vi "FreqStep-Init.vi"(0 "Fs (Hz)":dbl=100000.0, 1 "Npts":i32, 5 "delta f (Hz)":dbl=2000.0, 9 "Gate Control":T1(xcontrol)) -> (6 "omega_1":dbl[](array[numeric]), 10 "omega_2":dbl[](array[numeric]), 15 "delta Finst":dbl[](array[numeric]))   [LabVIEW 2015]
uses:
  Controls/Gate XCtl/Gate Control.xctl
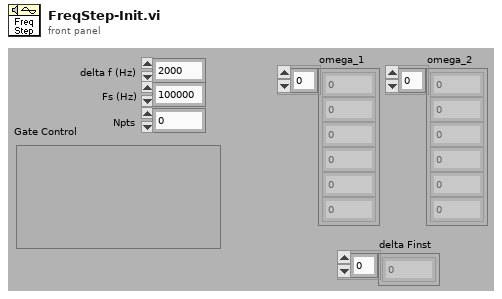
[diagram p1: front panel]
types:
  T1 = cluster{"Active":bool, "Delay (ms)":dbl, "Width (ms)":dbl, "Ramp (ms)":dbl}
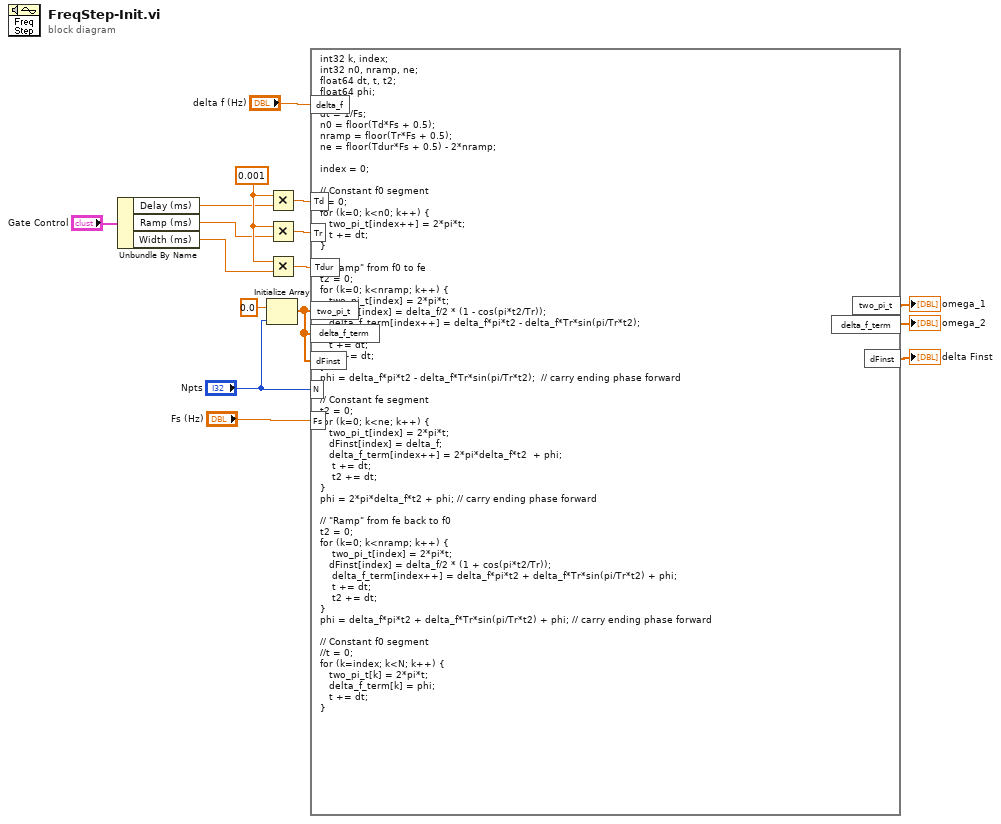
[diagram p0: block diagram]
diagram:
  w10 = 0.001 ("x")
  n1 = Unbundle By Name("Gate Control") -> ("Delay (ms)"=w5:dbl, "Ramp (ms)"=w4:dbl, "Width (ms)"=w3:dbl)
  n2 = Initialize Array(0.0 ("element"), "Npts") -> (w2:dbl[])
  n3 = Multiply(x=w10, y=w5) -> (x*y=w15:dbl)
  n4 = Multiply(x=w10, y=w4) -> (x*y=w14:dbl)
  n5 = Multiply(x=w10, y=w3) -> (x*y=w12:dbl)
  n6 = formula code="int32 k, index;\nint32 n0, nramp, ne;\nfloat64 dt, t, t2;\nfloat64 phi;\n\ndt = 1/Fs;\nn0 = floor(Td*Fs + 0.5);\nnramp = floor(Tr*Fs + 0.5);\nne = floor(Tdur*Fs + 0.5) - 2*nramp;\n\nindex = 0;\n\n// Constant f0 segment\nt = 0;\nfor (k=0; k<n0; k++) {\n   two_pi_t[index++] = 2*pi*t;\n   t += dt;\n}\n\n// \"Ramp\" from f0 to fe\nt2 = 0;\nfor (k=0; k<nramp; k++) {\n   two_pi_t[index] = 2*pi*t;\n   dFinst[index] = delta_f/2 * (1 - cos(pi*t2/Tr));\n   delta_f_term[index++] = delta_f*pi*t2 - delta_f*Tr*sin(pi/Tr*t2);\n\n   t += dt;\n   t2 += dt;\n}\nphi = delta_f*pi*t2 - delta_f*Tr*sin(pi/Tr*t2);  // carry ending phase forward\n\n// Constant fe segment\nt2 = 0;\nfor (k=0; k<ne; k++) {\n   two_pi_t[index] = 2*pi*t;\n   dFinst[index] = delta_f;\n   delta_f_term[index++] = 2*pi*delta_f*t2  + phi;\n    t += dt;\n    t2 += dt;\n}\nphi = 2*pi*delta_f*t2 + phi; // carry ending phase forward\n\n// \"Ramp\" from fe back to f0\nt2 = 0;\nfor (k=0; k<nramp; k++) {\n    two_pi_t[index] = 2*pi*t;\n   dFinst[index] = delta_f/2 * (1 + cos(pi*t2/Tr));\n    delta_f_term[index++] = delta_f*pi*t2 + delta_f*Tr*sin(pi/Tr*t2) + phi;\n    t += dt;\n    t2 += dt;\n}\nphi = delta_f*pi*t2 + delta_f*Tr*sin(pi/Tr*t2) + phi; // carry ending phase forward\n\n// Constant f0 segment\n//t = 0;\nfor (k=index; k<N; k++) {\n   two_pi_t[k] = 2*pi*t;\n   delta_f_term[k] = phi;\n   t += dt;\n}"("Fs"="Fs (Hz)", "Td"=w15, "two_pi_t"=w2, "Tr"=w14, "delta_f"="delta f (Hz)", "Tdur"=w12, "N"="Npts", "delta_f_term"=w2, "dFinst"=w2) -> ("two_pi_t"=→"omega_1":dbl[], "delta_f_term"=→"omega_2":dbl[], "dFinst"=→"delta Finst":dbl[])
